vi "Lens_Tuning_Login.vi"() -> ()   [LabVIEW 2018]
uses:
  Control/Control 4.ctl
  Sub_VI/Global Load.vi
panel:
  out "User Type":string
  out "Login":bool
  in  "User Name":string(combo)
  in  "Selection":string(combo)
  in  "Login":bool
  in  "Password":string
  in  "Vvdn Tech":bool
  in  "Stop Button":bool
  out "Date&Time":string
  out "error out":errorcluster
  in  "error in":errorcluster
  in  "Enum":T1
  in  "Login Credentials":T2={"User Name"=["Admin"], "User Password"=["admin"], "User Type 2"=[1]} {"User Type 2" items=["Administrator", "Operator", "QA"]}
  in  "Project-Name":string="LensTuning"
  in  "User Login":string
  # "USER LOGIN"
  # "Micrologic"
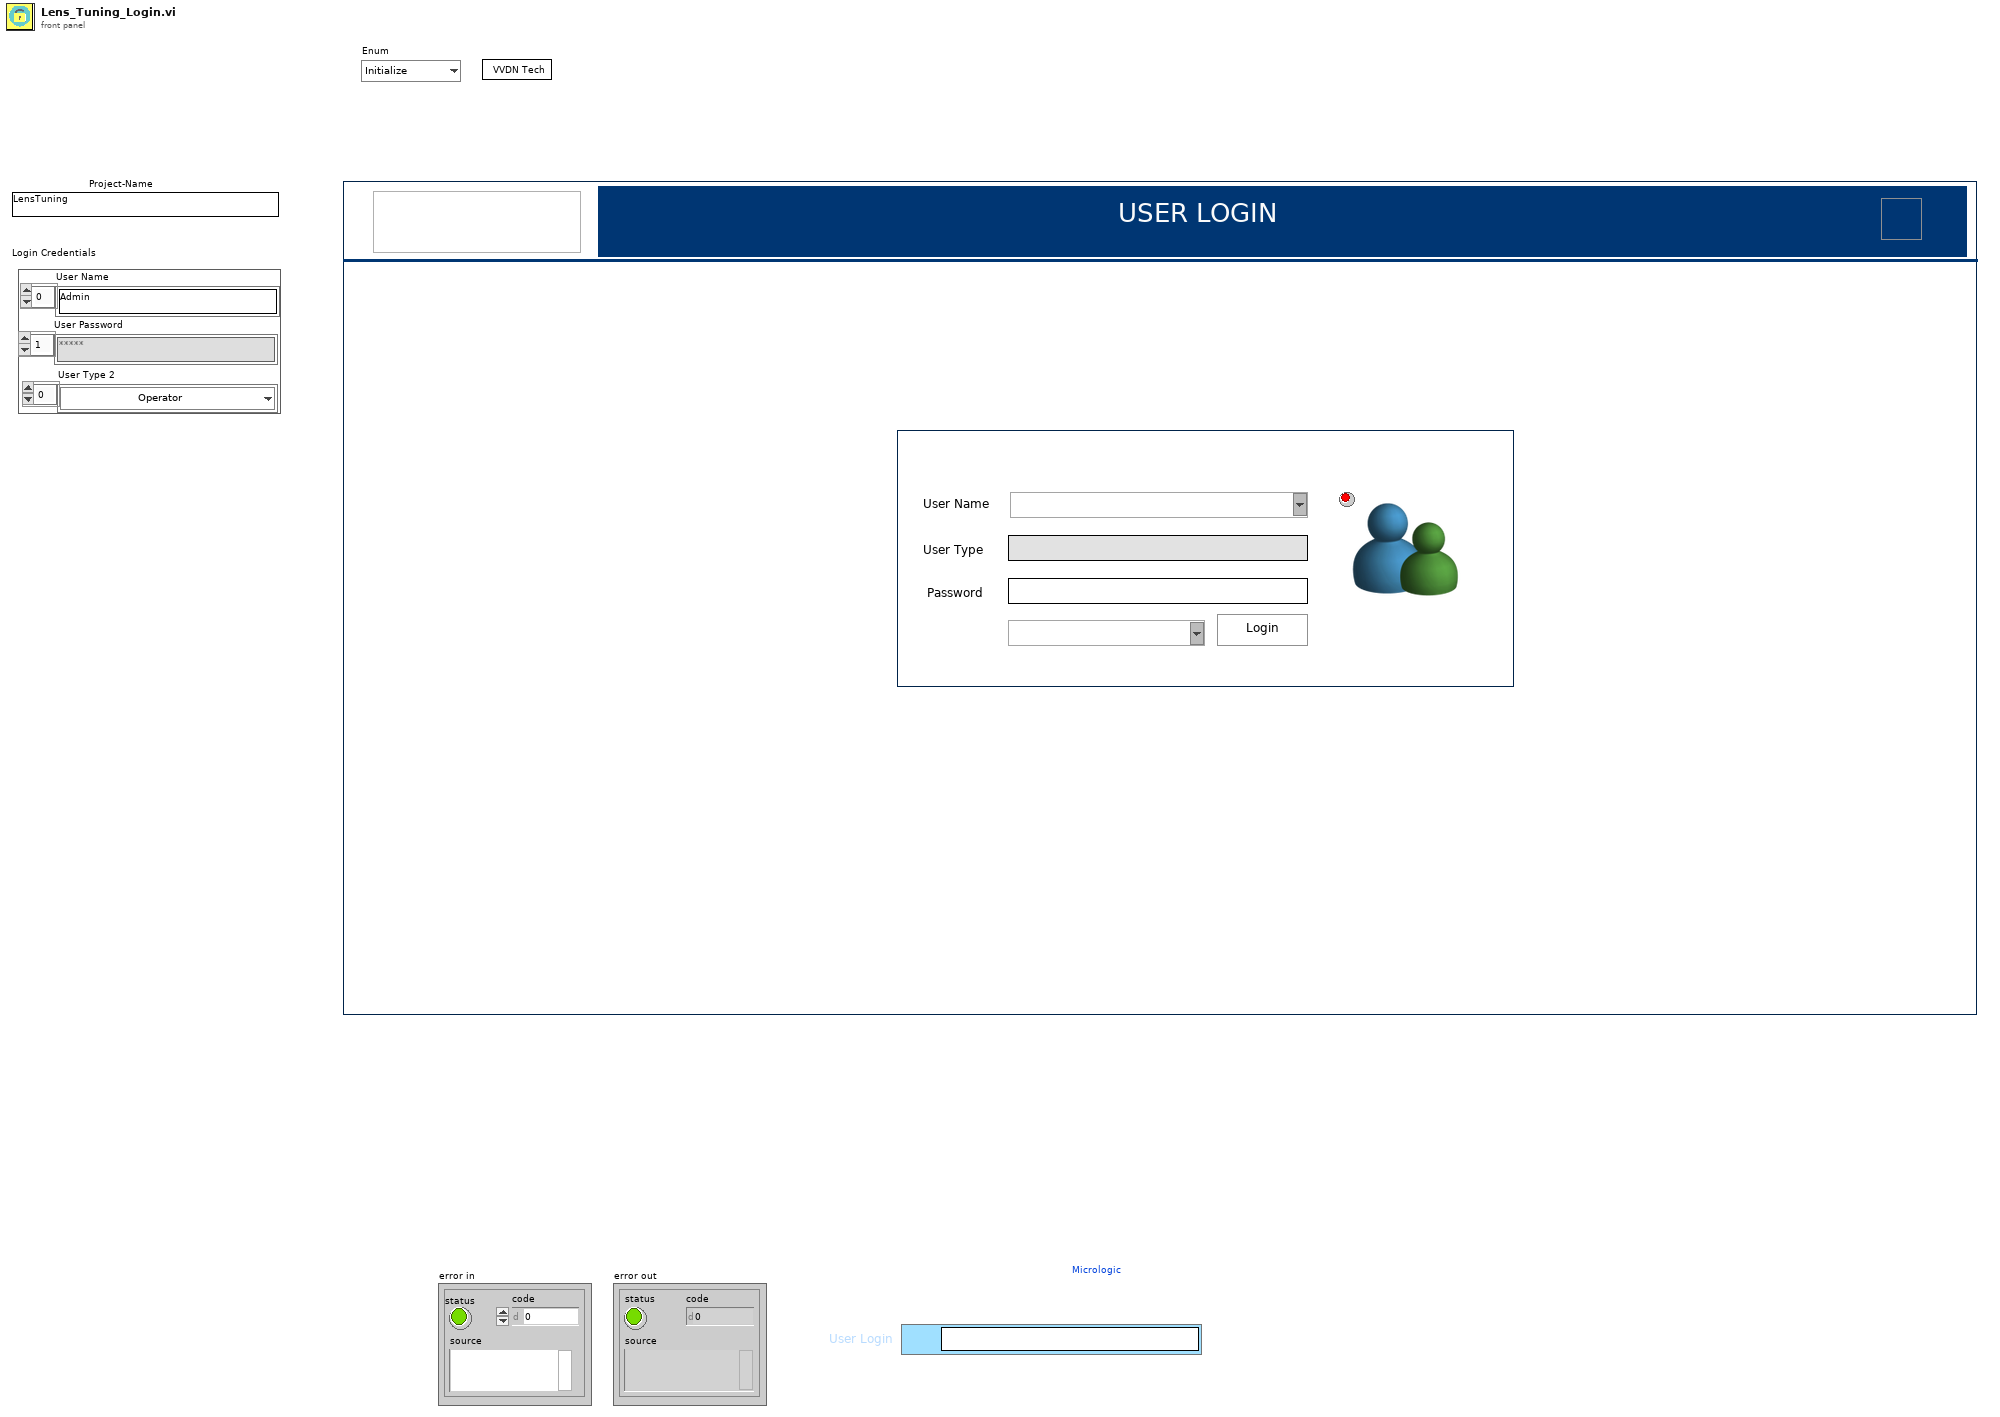
[diagram p1: front panel]
types:
  T1 = typedef "Control 4.ctl" = enum16{"Initialize", "Poll", "Login", "Cancel", "Exit"}
  T2 = cluster{"User Name":string[], "User Password":string[], "User Type 2":u16[]}
  T3 = cluster{"Default User ":string, "Default Password":string, "Default User Type":u16}[]
  T4 = enum32{"Invalid", "Standard", "Closed", "Hidden", "Minimized", "Maximized"}
  T5 = cluster{"User Login":string, "Password":string, "Default User Type":u16}
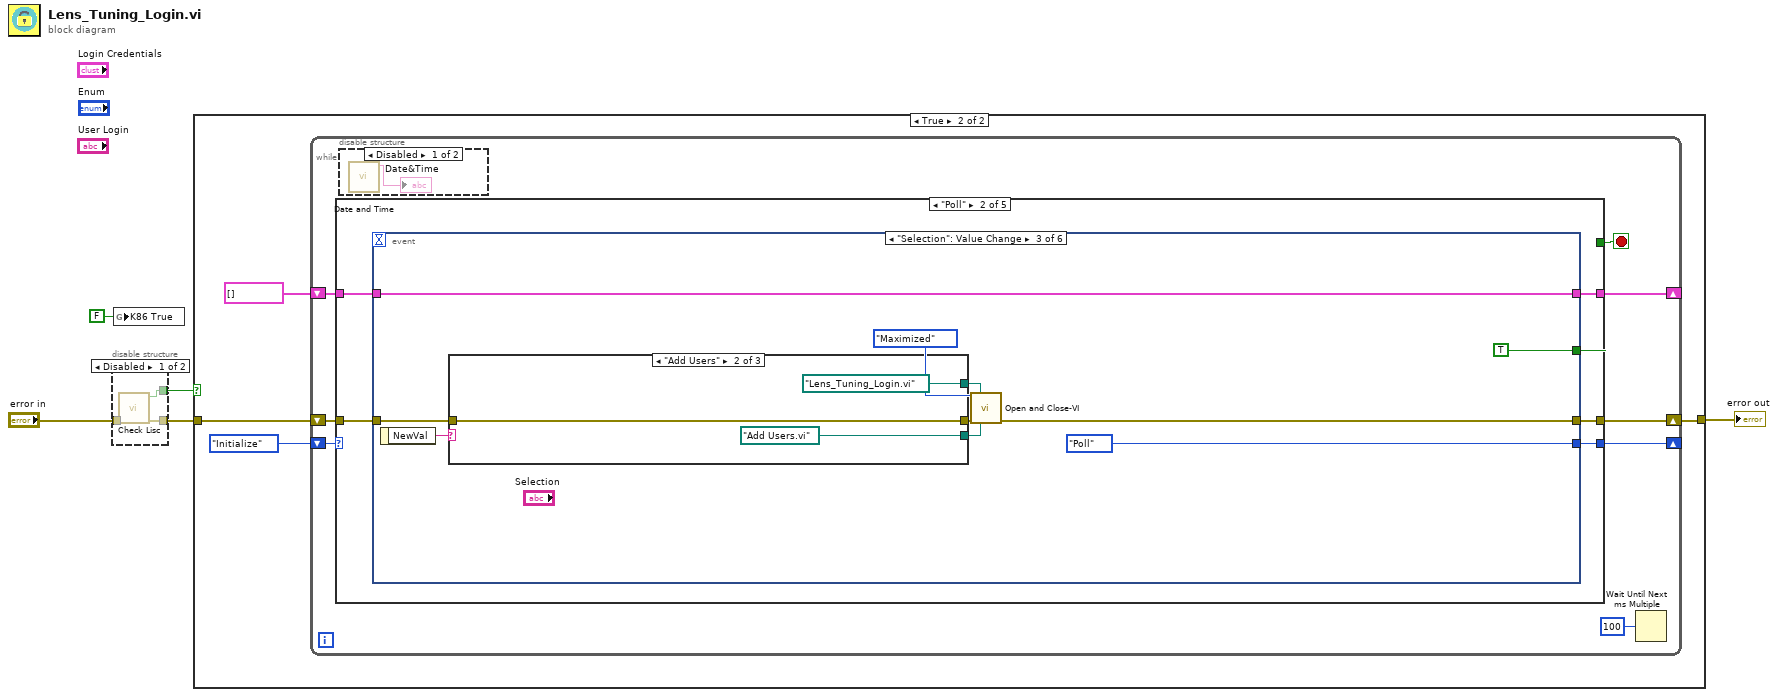
[diagram p0: block diagram]
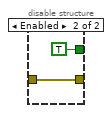
[diagram p2: hidden frame]
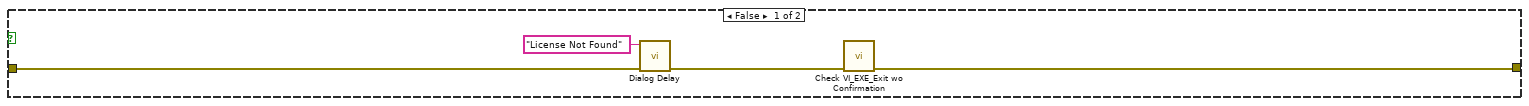
[diagram p3: hidden frame]
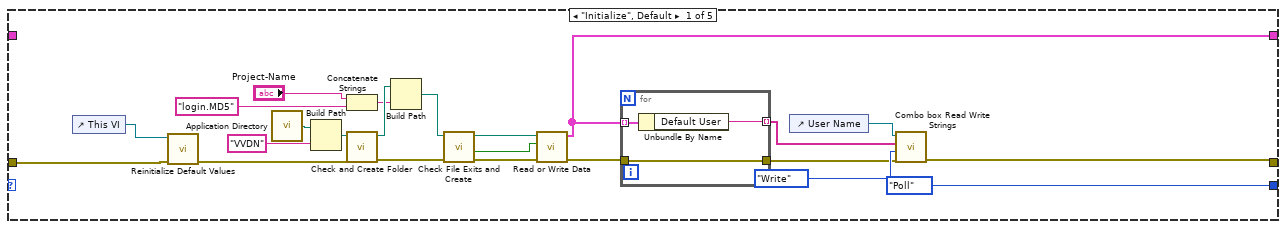
[diagram p5: hidden frame]
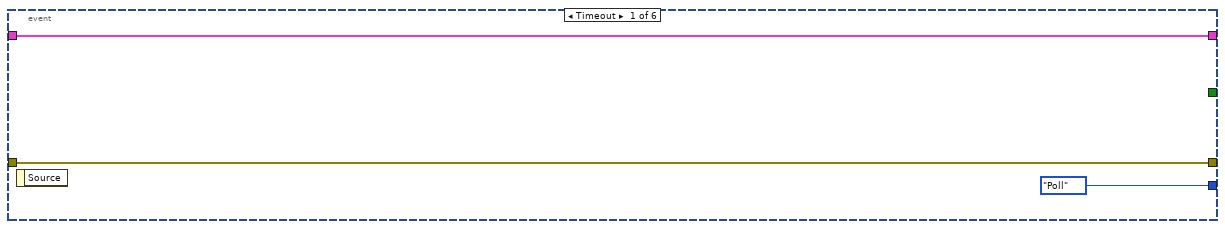
[diagram p6: hidden frame]
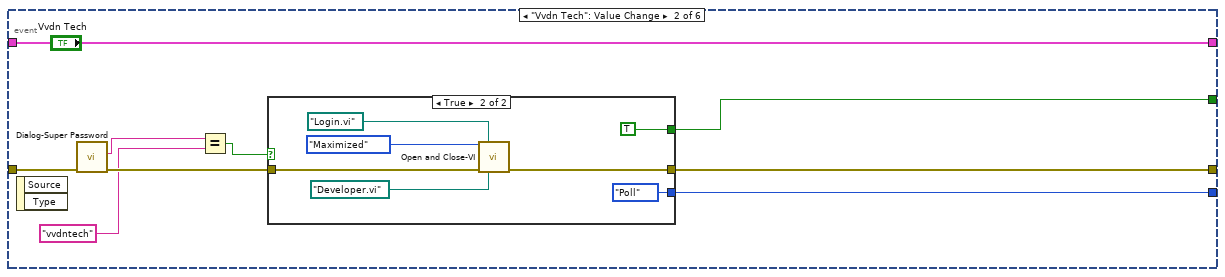
[diagram p7: hidden frame]
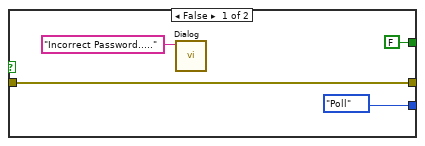
[diagram p8: hidden frame]
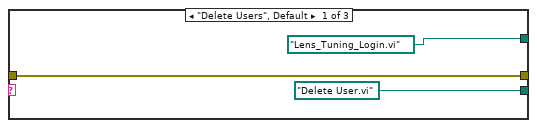
[diagram p9: hidden frame]
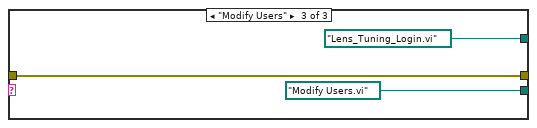
[diagram p10: hidden frame]
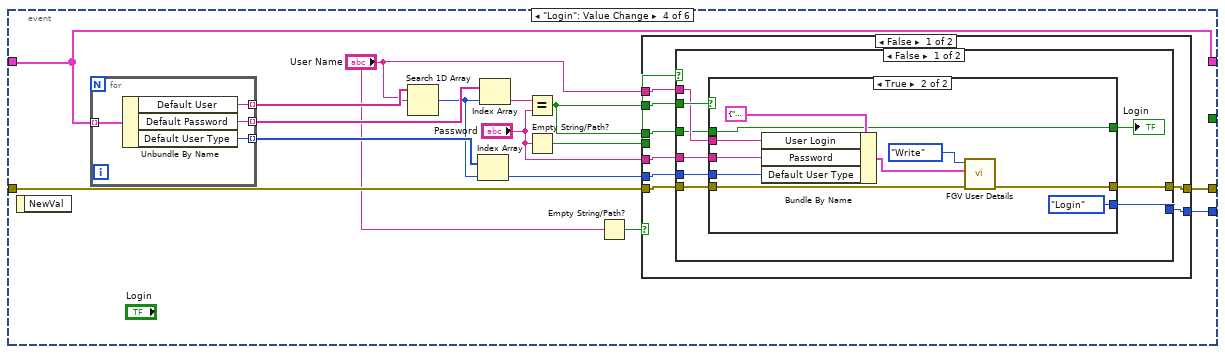
[diagram p11: hidden frame]
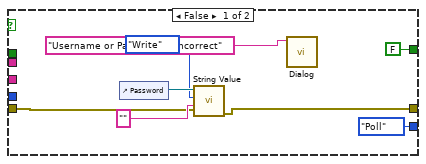
[diagram p12: hidden frame]
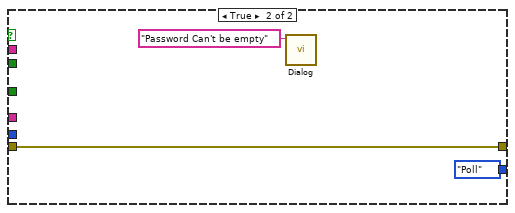
[diagram p13: hidden frame]
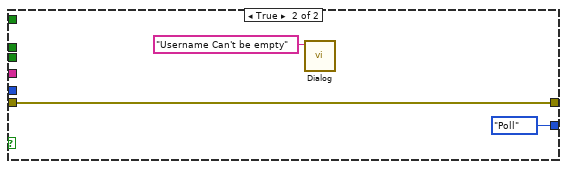
[diagram p14: hidden frame]
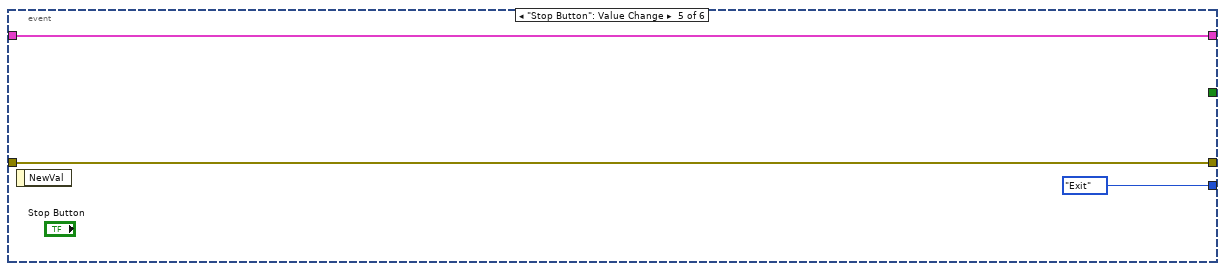
[diagram p15: hidden frame]
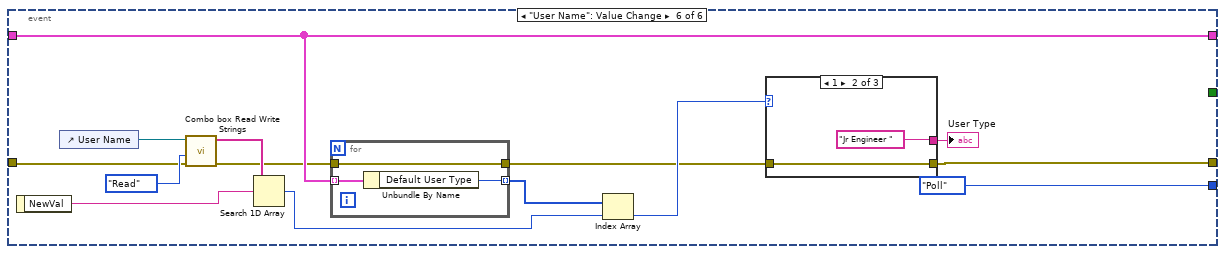
[diagram p16: hidden frame]
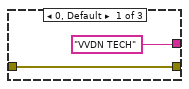
[diagram p17: hidden frame]
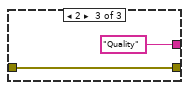
[diagram p18: hidden frame]
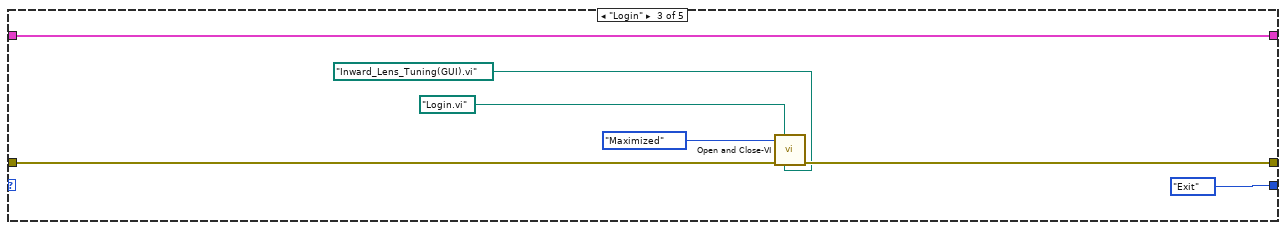
[diagram p19: hidden frame]
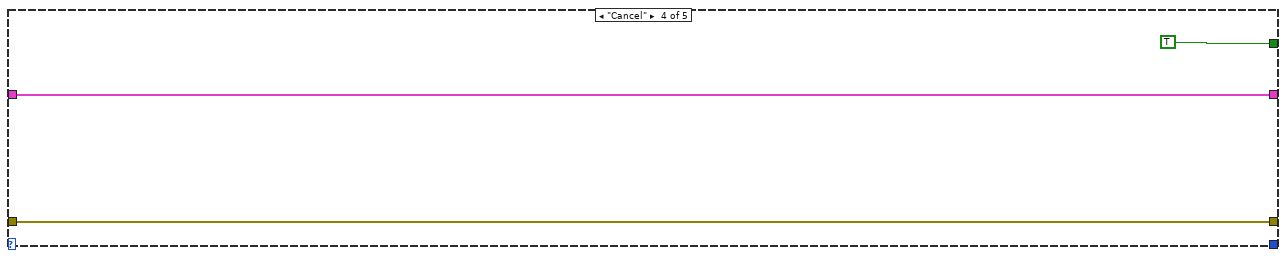
[diagram p20: hidden frame]
diagram:
  n1 = disable-structure shown="Disabled" {
    disable-tunnel: "error in" -> [w8 w9]
    disable-tunnel: [w7 w9] -> w3
    disable-tunnel: [w6 TRUE ("Lisc Found")] -> w2
    frame Disabled {
      n2 = call "Check Lisc.vi"("error in"=w8) -> ("error out"=w7:errorcluster, "Lisc Found"=w6:bool)  [unwired: 8 in, 1 out]
    }
    frame Enabled {
    }
  }
  n3 = global write "Global Load.vi" "K86 True"(FALSE ("K86 True")) -> ()
  n4 = case shown="True" w2 {
    tunnel: [w11 w17] -> w5
    tunnel: w3 -> [w14 w15]
    frame False {
      n5 = call "Dialog Delay.vi"("error in"=w14, "Status"="License Not Found") -> ("error out"=w12:errorcluster)  [unwired: 8 in, 1 out]
      n6 = call "Check VI_EXE_Exit wo Confirmation.vi"("error in"=w12) -> ("error out"=w11:errorcluster)  [unwired: 10 in]
    }
    frame True {
      n7 = while {
        shift-right: [w23] -> _
        shift-left: Control_4."Initialize" ("Enum") -> [w26]
        shift-right: [w24] -> _
        shift-left: T3 [] ("User Details") -> [w25]
        shift-right: [w21] -> w17
        shift-left: w15 -> [w22]
        stop <- w20 stop-if-true
        n8 = case shown="\"Poll\"" w26 {
          tunnel: w25 -> [_ w59 w195 w198 w208]
          tunnel: [w28 w58 w195 w198 w208] -> w24
          tunnel: [Control_4."Poll" ("Enum") w55 Control_4."Exit" ("Enum") _ Control_4."Exit" ("Enum")] -> w23
          tunnel: w22 -> [w35 w57 w193 w197 w204]
          tunnel: [w30 w56 w192 w197 w205] -> w21
          tunnel: [_ w54 _ TRUE TRUE] -> w20
          frame "Initialize", Default {
            n9 = control-ref of="This VI"() -> (w36:refnum<vi>)
            n10 = call "Reinitialize Default Values.vi"("error in (no error)"=w35, "VI in"=w36) -> ("error out"=w34:errorcluster)  [unwired: 9 in]
            n11 = call <vilib>:"Application Directory.vi"() -> ("Application Directory"=w47:path)
            n12 = Build Path(base path=w47, name or relative path="VVDN") -> (appended path=w43:path)
            n13 = Concatenate Strings("Project-Name", "login.MD5" ("string")) -> (w41:string)
            n14 = call "Check and Create Folder.vi"("error in (no error)"=w34, "Path In"=w43) -> ("error out"=w40:errorcluster, "Path Out"=w42:path)  [unwired: 7 in, 1 out]
            n15 = Build Path(base path=w42, name or relative path=w41) -> (appended path=w39:path)
            n16 = call "Check File Exits and Create.vi"("error in"=w40, "Path In"=w39) -> ("error out"=w48:errorcluster, "file exists?"=w50:bool, "Path Out"=w49:path)  [unwired: 6 in, 1 out]
            n17 = call "Read or Write Data.vi"("error in"=w48, "file exists?"=w50, "Path Out"=w49) -> ("error out"=w37:errorcluster, "User Details"=w28:T3)  [unwired: 7 in]
            n18 = for {
              tunnel: w28 -> [w53] mode=indexing
              tunnel: [w52] -> w29 mode=indexing
              tunnel: w37 -> [w51]
              tunnel: [w51] -> w31
              n19 = Unbundle By Name(w53) -> ("Default User"=w52:string)
            }
            n20 = control-ref of="User Name"() -> (w33:refnum<vi>)
            n21 = call "Combo box Read Write Strings.vi"("error in (no error)"=w31, "Enum"=enum16{"Read", "Write"}."Write", "Strings []"=w29, "ComboBox in"=w33) -> ("error out"=w30:errorcluster)  [unwired: 6 in, 1 out]
          }
          frame "Poll" {
            n22 = event shown="[2] \"Selection\": Value Change" {
              selector: _ -> [_ _ _ _ _ _]
              dyn-events: _ -> [_ _ _ _ _ _]
              timeout: _ -> [_ _ _ _ _ _]
              tunnel: w59 -> [w62 w71 w90 w102 w164 w177]
              tunnel: [w62 w71 w90 w102 w164 w177] -> w58
              tunnel: w57 -> [w61 w66 w87 w108 w165 w167]
              tunnel: [w61 w70 w91 w107 w165 w171] -> w56
              tunnel: [Control_4."Poll" ("Enum") w67 Control_4."Poll" ("Enum") w106 Control_4."Exit" ("Enum") Control_4."Poll" ("Enum")] -> w55
              tunnel: [_ w68 TRUE _ _ _] -> w54
              event Timeout {
                n23 = event-data() -> ()  [unwired: 1 in, 1 out]
              }
              event "Vvdn Tech": Value Change {
                n24 = event-data() -> ()  [unwired: 1 in, 2 out]
                n25 = call "Dialog-Super Password.vi"("error in"=w66) -> ("error out"=w65:errorcluster, "Password Out"=w64:string)  [unwired: 8 in, 1 out]
                n26 = Equal?(x=w64, y="vvdntech") -> (x = y?=w69:bool)
                n27 = case shown="True" w69 {
                  tunnel: w65 -> [w75 w79]
                  tunnel: [w75 w78] -> w70
                  tunnel: [FALSE TRUE] -> w68
                  tunnel: [Control_4."Poll" ("Enum") Control_4."Poll" ("Enum")] -> w67
                  frame False {
                    n28 = call "Dialog.vi"("Status"="Incorrect Password.....") -> ()  [unwired: 10 in, 1 out]
                  }
                  frame True {
                    n29 = call "Open and Close-VI.vi"("State"=T4."Maximized", "Close VI"=path "Login.vi", "error in"=w79, "Open VI"=path "Developer.vi") -> ("error out"=w78:errorcluster)  [unwired: 11 in]
                  }
                }
              }
              event "Selection": Value Change {
                n30 = event-data() -> ("NewVal"=w92:string)  [unwired: 1 in]
                n31 = case shown="\"Add Users\"" w92 {
                  tunnel: [path "Lens_Tuning_Login.vi" path "Lens_Tuning_Login.vi" path "Lens_Tuning_Login.vi"] -> w85
                  tunnel: [path "Delete User.vi" path "Add Users.vi" path "Modify Users.vi"] -> w84
                  tunnel: w87 -> [w93 w96 w99]
                  tunnel: [w93 w96 w99] -> w83
                  frame "Delete Users", Default {
                  }
                  frame "Add Users" {
                  }
                  frame "Modify Users" {
                  }
                }
                n32 = call "Open and Close-VI.vi"("State"=T4."Maximized", "Close VI"=w85, "error in"=w83, "Open VI"=w84) -> ("error out"=w91:errorcluster)  [unwired: 11 in]
              }
              event "Login": Value Change {
                n33 = event-data() -> ()  [unwired: 1 in, 1 out]
                n34 = for {
                  tunnel: w102 -> [w162] mode=indexing
                  tunnel: [w161] -> w115 mode=indexing
                  tunnel: [w160] -> w114 mode=indexing
                  tunnel: [w159] -> w112 mode=indexing
                  n35 = Unbundle By Name(w162) -> ("Default User"=w161:string, "Default Password"=w160:string, "Default User Type"=w159:u16)
                }
                n36 = Search 1D Array(1D array=w115, element="User Name") -> (index of element=w111:i32)  [unwired: 1 in]
                n37 = Index Array(array=w112, index=w111) -> (element=w110:u16)
                n38 = Index Array(array=w114, index=w111) -> (element=w113:string)
                n39 = Equal?(x=w113, y="Password") -> (x = y?=w103:bool)
                n40 = Empty String/Path?(string/path="Password") -> (empty?=w116:bool)
                n41 = Empty String/Path?(string/path="User Name") -> (empty?=w104:bool)
                n42 = case shown="False" w104 {
                  tunnel: w116 -> [w125 _]
                  tunnel: w103 -> [w124 _]
                  tunnel: w110 -> [w123 _]
                  tunnel: "User Name" -> [w122 _]
                  tunnel: "Password" -> [w121 _]
                  tunnel: w108 -> [w120 w158]
                  tunnel: [w119 w158] -> w107
                  tunnel: [w118 Control_4."Poll" ("Enum")] -> w106
                  tunnel: w103 -> [w117 _]
                  frame False {
                    n43 = case shown="False" w125 {
                      tunnel: [w134 Control_4."Poll" ("Enum")] -> w118
                      tunnel: w124 -> [w133 _]
                      tunnel: w123 -> [w132 _]
                      tunnel: w122 -> [w131 _]
                      tunnel: w121 -> [w130 _]
                      tunnel: w120 -> [w129 w153]
                      tunnel: [w128 w153] -> w119
                      tunnel: w117 -> [w127 _]
                      frame False {
                        n44 = case shown="True" w133 {
                          tunnel: [Control_4."Poll" ("Enum") Control_4."Login" ("Enum")] -> w134
                          tunnel: w132 -> [_ w148]
                          tunnel: w131 -> [_ w150]
                          tunnel: w130 -> [_ w149]
                          tunnel: w129 -> [w135 w145]
                          tunnel: [w136 w144] -> w128
                          tunnel: w127 -> [_ w143]
                          tunnel: [FALSE w143] -> w126
                          frame False {
                            n45 = control-ref of="Password"() -> (w139:refnum<vi>)
                            n46 = call "String Value.vi"("error in"=w135, "String In"="", "Read/Write"=enum16{"Write", "Read"}."Write", "String in"=w139) -> ("error out"=w136:errorcluster)  [unwired: 6 in, 1 out]
                            n47 = call "Dialog.vi"("Status"="Username or Password is Incorrect") -> ()  [unwired: 10 in, 1 out]
                          }
                          frame True {
                            n48 = Bundle By Name(cluster=T5 {"User Login"="", "Password"="", "Default User Type"=0} ("output cluster"), "User Login"=w150, "Password"=w149, "Default User Type"=w148) -> (w147:T5)
                            n49 = call "FGV User Details.vi"("error in"=w145, "User Details"=w147, "Action"=enum16{"Initialize", "Read", "Write"}."Write") -> ("error out"=w144:errorcluster)  [unwired: 7 in, 1 out]
                          }
                        }
                        "Login" <- w126
                      }
                      frame True {
                        n50 = call "Dialog.vi"("Status"="Password Can't be empty") -> ()  [unwired: 10 in, 1 out]
                      }
                    }
                  }
                  frame True {
                    n51 = call "Dialog.vi"("Status"="Username Can't be empty") -> ()  [unwired: 10 in, 1 out]
                  }
                }
              }
              event "Stop Button": Value Change {
                n52 = event-data() -> ()  [unwired: 1 in, 1 out]
              }
              event "User Name": Value Change {
                n53 = event-data() -> ("NewVal"=w178:string)  [unwired: 1 in]
                n54 = control-ref of="User Name"() -> (w170:refnum<vi>)
                n55 = call "Combo box Read Write Strings.vi"("error in (no error)"=w167, "Enum"=enum16{"Read", "Write"}."Read", "ComboBox in"=w170) -> ("error out"=w166:errorcluster, "Strings[]Out"=w168:string[])  [unwired: 7 in]
                n56 = Search 1D Array(1D array=w168, element=w178) -> (index of element=w175:i32)  [unwired: 1 in]
                n57 = for {
                  tunnel: w177 -> [w188] mode=indexing
                  tunnel: [w187] -> w176 mode=indexing
                  tunnel: w166 -> [w186]
                  tunnel: [w186] -> w172
                  n58 = Unbundle By Name(w188) -> ("Default User Type"=w187:u16)
                }
                n59 = Index Array(array=w176, index=w175) -> (element=w174:u16)
                n60 = case shown="1" w174 {
                  tunnel: ["VVDN TECH" ("User Type") "Jr Engineer " ("User Type") "Quality" ("User Type")] -> w173
                  tunnel: w172 -> [w180 w182 w184]
                  tunnel: [w180 w182 w184] -> w171
                  frame 0, Default {
                  }
                  frame 1 {
                  }
                  frame 2 {
                  }
                }
                "User Type" <- w173
              }
            }
          }
          frame "Login" {
            n61 = call "Open and Close-VI.vi"("State"=T4."Maximized", "Close VI"=path "Login.vi", "error in"=w193, "Open VI"=path "Inward_Lens_Tuning(GUI).vi") -> ("error out"=w192:errorcluster)  [unwired: 11 in]
          }
          frame "Cancel" {
          }
          frame "Exit" {
            n62 = control-ref of="This VI"() -> (w203:refnum<vi>)
            n63 = invoke class="VI" method="FP.Close"(reference=w203, error in=w204) -> (reference out=w199:refnum<vi>, error out=w201:errorcluster)  [unwired: 1 in, 1 out]
            n64 = Close Reference(reference=w199, error in (no error)=w201) -> (error out=w200:errorcluster)
            n65 = call <vilib>:"Clear Errors.vi"("error in (no error)"=w200) -> ("error out"=w202:errorcluster)  [unwired: 5 in, 1 out]
            n66 = call "Check VI_EXE_Exit wo Confirmation.vi"("error in"=w202) -> ("error out"=w205:errorcluster)  [unwired: 10 in]
          }
        }
        n67 = disable-structure shown="Disabled" {
          frame Disabled {
            n68 = call "Date and Time.vi"() -> ("date string"=→"Date&Time":string)  [unwired: 11 in]
          }
          frame Enabled {
          }
        }
        n69 = Wait Until Next ms Multiple(millisecond multiple=u32 100) -> ()  [unwired: 1 out]
      }
    }
  }
  "error out" <- w5
